vi "AC Couple (1 Ch SGL Array No Window).vi"(8 "error in (no error)":errorcluster, 10 "Signal":sgl[](array[numeric])) -> (0 "error out":errorcluster, 1 "DC":sgl, 2 "AC Coupled":sgl[](array[numeric]))   [LabVIEW 2017, in "VibrationAnalysisFunctions.lvlib"]
uses:
  <vilib>/addons/InsightCM/Utilities/Analysis/Vibration/VibrationAnalysisFunctions.lvlib
  <vilib>/Analysis/baseanly.llb/Mean (DBL).vi
  <vilib>/Analysis/NI_AALBase.lvlib
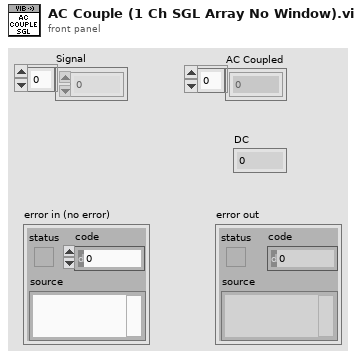
[diagram p1: front panel]
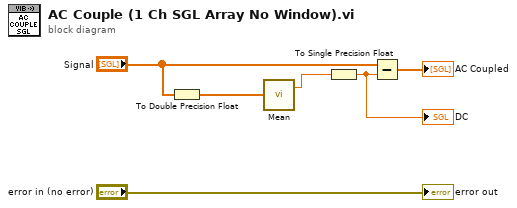
[diagram p0: block diagram]
diagram:
  n1 = To Double Precision Float(number="Signal") -> (double precision float=w1:dbl[])
  n2 = call-poly <vilib>:"Mean.vi"("X"=w1) -> ("mean"=w3:dbl)  [unwired: 1 out]
  n3 = To Single Precision Float(number=w3) -> (single precision float=w2:sgl)
  "DC" <- w2
  n4 = Subtract(x="Signal", y=w2) -> (x-y=→"AC Coupled":sgl[])
  "error out" <- "error in (no error)"
